vi "9207_two-channel_readout.vi"() -> ()   [LabVIEW 2018]
uses:
  <vilib>/DAQmx/read.llb/DAQmx Read (Analog 1D DBL NChan 1Samp).vi
  <vilib>/DAQmx/create/channels.llb/DAQmx Create Channel (AI-Voltage-Basic).vi
  <vilib>/DAQmx/miscellaneous.llb/DAQmx Fill In Error Info.vi
panel:
  in  "9207 ch1":tag
  out "All":dbl[][](array[numeric])
  out "Latest":dbl[](array[numeric]) format="%0.2f"
  out "error out":errorcluster
  in  "stop":bool
  in  "9207 Ch0":tag
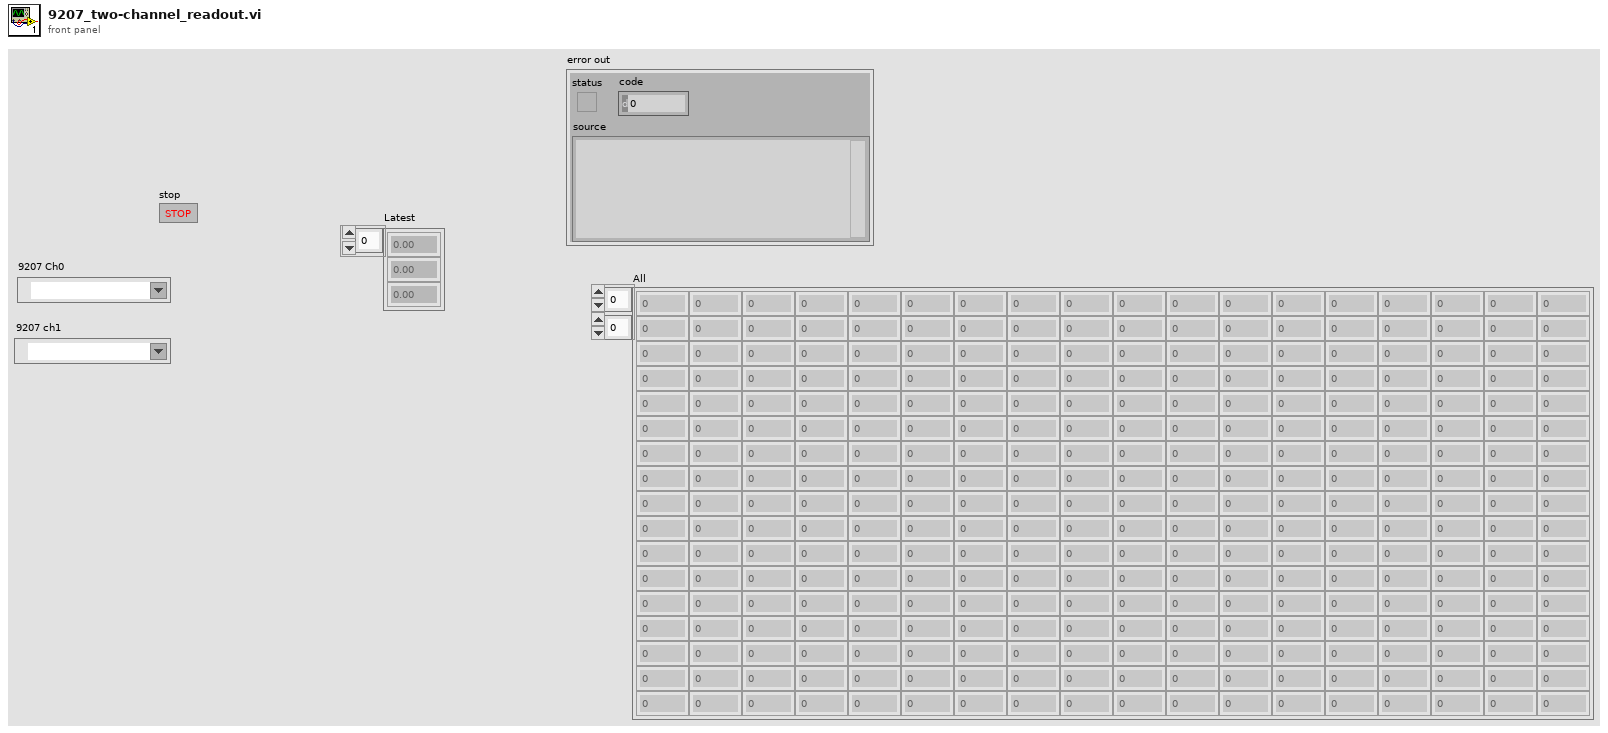
[diagram p1: front panel]
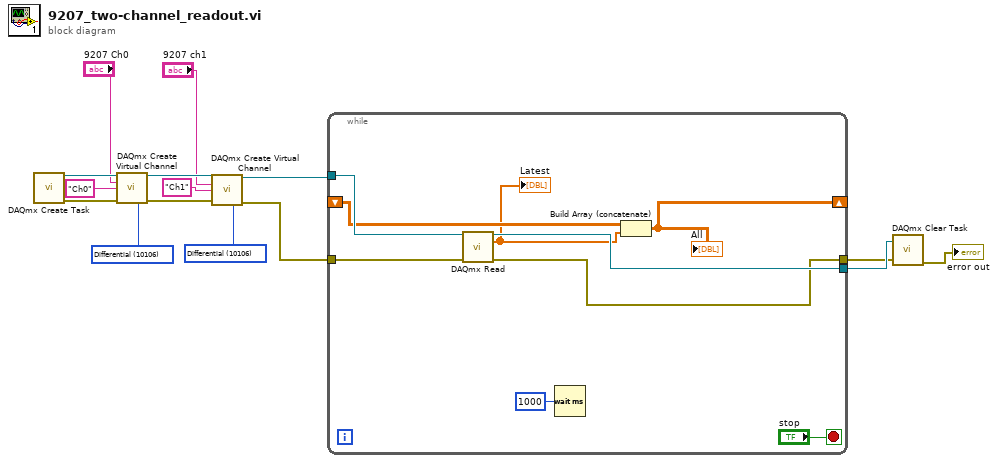
[diagram p0: block diagram]
diagram:
  w1 = 10106 items=["Default"=-1, "RSE"=10083, "NRSE"=10078, "Differential"=10106, "Pseudodifferential"=12529] ("input terminal configuration")
  w12 = 10106 items=["Default"=-1, "RSE"=10083, "NRSE"=10078, "Differential"=10106, "Pseudodifferential"=12529] ("input terminal configuration")
  n1 = call <vilib>:"DAQmx Create Task.vi"() -> ("task out"=w15:refnum<k21>, "error out"=w14:errorcluster)  [unwired: 14 in]
  n2 = call-poly <vilib>:"DAQmx Create Virtual Channel.vi"("task in"=w15, "input terminal configuration"=w12, "physical channels"="9207 Ch0", "name to assign"="Ch0", "error in"=w14) -> ("task out"=w7:refnum<k21>, "error out"=w6:errorcluster)  [unwired: 9 in]
  n3 = call-poly <vilib>:"DAQmx Create Virtual Channel.vi"("task in"=w7, "input terminal configuration"=w1, "physical channels"="9207 ch1", "name to assign"="Ch1", "error in"=w6) -> ("task out"=w3:refnum<k21>, "error out"=w2:errorcluster)  [unwired: 9 in]
  n4 = while {
    tunnel: w3 -> [w24]
    tunnel: w2 -> [w23]
    shift-right: [w16] -> _
    shift-left: _ -> [w20]
    tunnel: [w19] -> w11
    tunnel: [w18] -> w10
    stop <- "stop" stop-if-true
    n5 = call-poly <vilib>:"DAQmx Read.vi"("task/channels in"=w24, "error in"=w23) -> ("task out"=w19:refnum<k21>, "data"=w17:dbl[], "error out"=w18:errorcluster)  [unwired: 11 in]
    "Latest" <- w17
    n6 = Wait (ms)(milliseconds to wait=u32 1000) -> ()  [unwired: 1 out]
    n7 = Build Array (concatenate)(w20, w17) -> (w16:dbl[][])
    "All" <- w16
  }
  n8 = call <vilib>:"DAQmx Clear Task.vi"("task in"=w11, "error in"=w10) -> ("error out"=→"error out":errorcluster)  [unwired: 13 in]
